vi "BuildFileListFile.vi"(10 "Task":enum16{"BuildFile", "ReadFile"}(ring)=enum."ReadFile") -> (0 "error out":errorcluster, 3 "Instruments":cluster{"Folder Path":path, "tags":string[]}[](array[cluster]))   [LabVIEW 2022 SP3]
uses:
  Mic/Mic_Global.vi
panel:
  out "text":string
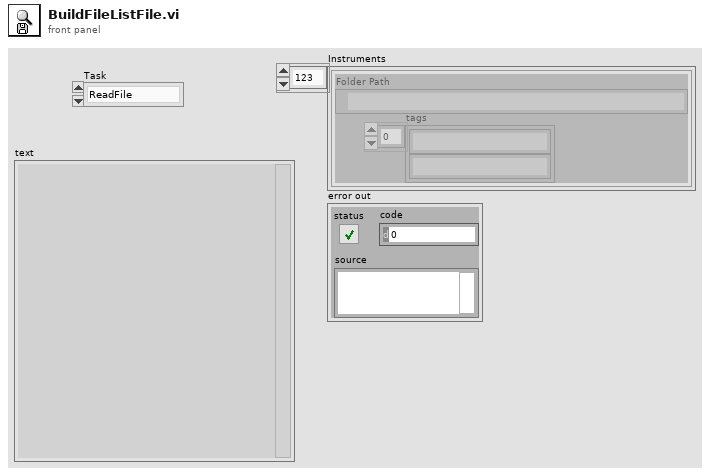
[diagram p1: front panel]
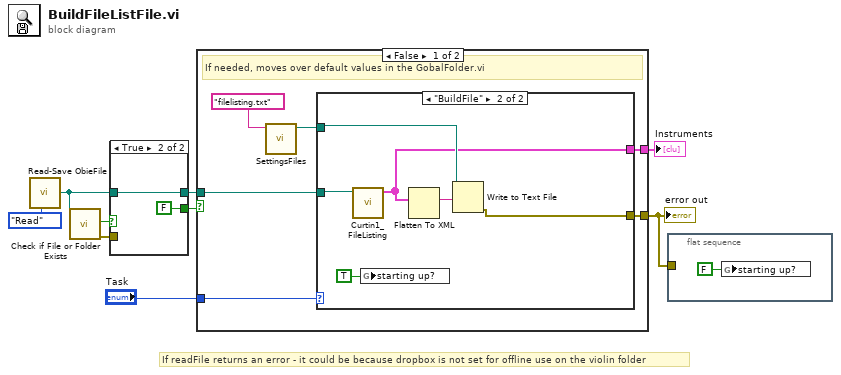
[diagram p0: block diagram]
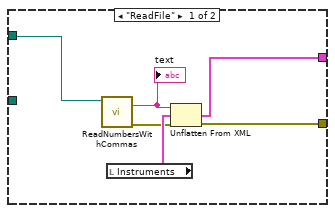
[diagram p2: hidden frame]
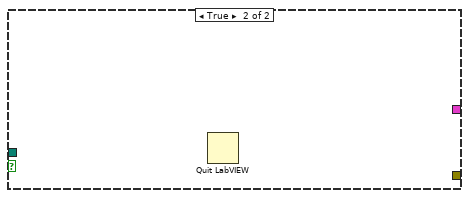
[diagram p3: hidden frame]
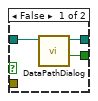
[diagram p4: hidden frame]
diagram:
  # "If readFile returns an error - it could be because dropbox is not set for offline use on the violin folder"
  n1 = call "Read-Save ObieFile.vi"("Task"=enum16{"Save", "Read"}."Read") -> ("DataPath Out"=w6:path)  [unwired: 8 in, 2 out]
  n2 = call <vilib>:"Check if File or Folder Exists.vi"("path"=w6) -> ("error out"=w2:errorcluster, "file or folder exists?"=w7:bool)  [unwired: 8 in, 1 out]
  n3 = case shown="True" w7 {
    tunnel: w6 -> [w12 w14]
    tunnel: [w11 w14] -> w4
    tunnel: [w10 FALSE ("canceled?")] -> w3
    tunnel: w2 -> [_ _]
    frame False {
      n4 = call "DataPathDialog.vi"("Path"=w12) -> ("canceled?"=w10:bool, "Path out"=w11:path)  [unwired: 9 in]
    }
    frame True {
    }
  }
  n5 = case shown="False" w3 {
    tunnel: [w20 _] -> w1
    tunnel: "Task" -> [w19 _]
    tunnel: [w18 _] -> w8
    tunnel: w4 -> [w17 _]
    frame False {
      # "If needed, moves over default values in the GobalFolder.vi"
      n6 = call "SettingsFiles.vi"("settings file name"="filelisting.txt" ("name or relative path")) -> ("file path"=w15:path)  [unwired: 9 in, 1 out]
      n7 = case shown="\"BuildFile\"" w19 {
        tunnel: w15 -> [w23 w32]
        tunnel: [w26 w28] -> w20
        tunnel: [w24 w31] -> w18
        tunnel: w17 -> [_ w29]
        frame "ReadFile" {
          n8 = call "ReadNumbersWithCommas.vi"("file (use dialog)"=w23) -> ("error out"=w21:errorcluster, "text"=w22:string)  [unwired: 7 in, 2 out]
          "text" <- w22
          n9 = local read "Instruments"() -> (w25:cluster{"Folder Path":path, "tags":string[]}[])
          n10 = Unflatten From XML(xml string=w22, type=w25, error in (no error)=w21) -> (value=w24:cluster{"Folder Path":path, "tags":string[]}[], error out=w26:errorcluster)
        }
        frame "BuildFile" {
          n11 = call "Curtin1_FileListing.vi"("Folder Path"=w29) -> ("Array"=w31:cluster{"Folder Path":path, "tags":string[]}[])  [unwired: 10 in]
          n12 = global write "Mic_Global.vi" "starting up?"(TRUE ("starting up?")) -> ()
          n13 = Flatten To XML(6:w31) -> (2:w30:string)
          n14 = Write to Text File(file (use dialog)=w32, text=w30) -> (error out=w28:errorcluster)  [unwired: 2 in, 2 out]
        }
      }
    }
    frame True {
      n15 = Quit LabVIEW() -> ()  [unwired: 1 in]
    }
  }
  "error out" <- w1
  "Instruments" <- w8
  n16 = flat-sequence {
    tunnel: w1 -> [_]
    frame #0 {
      n17 = global write "Mic_Global.vi" "starting up?"(FALSE ("starting up?")) -> ()
    }
  }
